vi "VI Control Enable.vi"(6 "Enable List":string[](array[string]), 7 "Disable List":string[](array[string]), 11 "VI引用句柄":refnum<vi>) -> ()   [LabVIEW 2018, in "CAN FD.lvlib"]
uses:
  CAN FD.lvlib
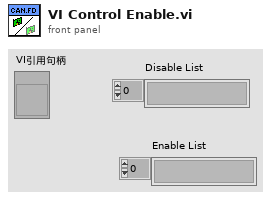
[diagram p1: front panel]
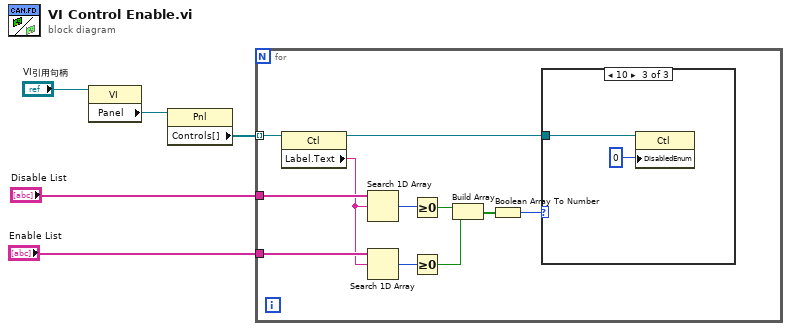
[diagram p0: block diagram]
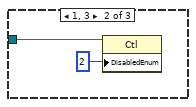
[diagram p3: hidden frame]
diagram:
  n1 = property class="VI"(reference="VI引用句柄") -> ("Panel"=w4:refnum<vi>)  [unwired: 1 in, 2 out]
  n2 = property class="Pnl"(reference=w4) -> ("Controls[]"=w3:refnum<vi>[])  [unwired: 1 in, 2 out]
  n3 = for {
    tunnel: w3 -> [w16] mode=indexing
    tunnel: "Disable List" -> [w15]
    tunnel: "Enable List" -> [w14]
    n4 = property class="Ctl"(reference=w16) -> (reference out=w6:refnum<vi>, "Label.Text"=w13:string)  [unwired: 1 in, 1 out]
    n5 = Search 1D Array(1D array=w15, element=w13) -> (index of element=w12:i32)  [unwired: 1 in]
    n6 = Search 1D Array(1D array=w14, element=w13) -> (index of element=w11:i32)  [unwired: 1 in]
    n7 = Greater Or Equal To 0?(x=w12) -> (x >= 0?=w10:bool)
    n8 = Greater Or Equal To 0?(x=w11) -> (x >= 0?=w9:bool)
    n9 = Build Array(w10, w9) -> (w8:bool[])
    n10 = Boolean Array To Number(Boolean array=w8) -> (number=w7:u32)
    n11 = case shown="10" w7 {
      tunnel: w6 -> [_ w18 w20]
      frame 0, Default {
      }
      frame 1, 3 {
        n12 = property class="Ctl"(reference=w18, "DisabledEnum"=2) -> ()  [unwired: 1 in, 2 out]
      }
      frame 2 {
        n13 = property class="Ctl"(reference=w20, "DisabledEnum"=0) -> ()  [unwired: 1 in, 2 out]
      }
    }
  }
